vi "Create Connections.vi"(8 "error in (no error)":errorcluster, 11 "RT Data Cluster in":T1={"Timekeeper hdl"="", "clkDisc session"=variant, "Compiled Data"={"SyncMod?"=FALSE, "SyncMod"="", "ConnectionSettings"={"Mode"=enum."Generate sample clock", "pxitrig"=FALSE, "pfi0"=FALSE, "pfi1"=FALSE, "pfi2"=FALSE, "External Pin"=enum."PFI0", "Routes"=[]}, "TimeKeeper"="", "ScanOffset(%)"=0.0, "StartDelay(s)"=0, "Time Ref Settings"={"Time Reference"=enum."GPS", "Priority 1"=0, "Priority 2"=0, "IRIG type"=enum."IRIGB AM", "Terminal"="", "PPSSetTime"=FALSE, "Start Time"=timestamp(0 s since 1904-01-01)}, "FIFO Locations"={"BoardTime"=[], "Status"=[]}}, "OutputsData"=[], "OutputsFIFO"=refnum, "Scan Period"=0, "Timekeeper type"=enum."6683", "SyncMod type"=enum."6683", "SyncMod hdl"="", "Custom Device Name"=""} {"Compiled Data"."Time Ref Settings"."Priority 2" min=0 max=255; "Compiled Data"."Time Ref Settings"."Priority 1" min=0 max=255}) -> (0 "error out":errorcluster, 3 "RT Data Cluster out":T1={"Timekeeper hdl"="", "clkDisc session"=variant, "Compiled Data"={"SyncMod?"=FALSE, "SyncMod"="", "ConnectionSettings"={"Mode"=enum."Generate sample clock", "pxitrig"=FALSE, "pfi0"=FALSE, "pfi1"=FALSE, "pfi2"=FALSE, "External Pin"=enum."PFI0", "Routes"=[]}, "TimeKeeper"="", "ScanOffset(%)"=0.0, "StartDelay(s)"=0, "Time Ref Settings"={"Time Reference"=enum."GPS", "Priority 1"=0, "Priority 2"=0, "IRIG type"=enum."IRIGB AM", "Terminal"="", "PPSSetTime"=FALSE, "Start Time"=timestamp(0 s since 1904-01-01)}, "FIFO Locations"={"BoardTime"=[], "Status"=[]}}, "OutputsData"=[], "OutputsFIFO"=refnum, "Scan Period"=0, "Timekeeper type"=enum."6683", "SyncMod type"=enum."6683", "SyncMod hdl"="", "Custom Device Name"=""} {"Compiled Data"."Time Ref Settings"."Priority 2" min=0 max=255; "Compiled Data"."Time Ref Settings"."Priority 1" min=0 max=255})   [LabVIEW 2020, in "NI Synchronization Engine.lvlib"]
uses:
  NI Synchronization Engine.lvlib
  Timekeeper Route Pin.ctl
  <instrlib>/niSync/niSync.llb/niSync Create Clock (Frequency).vi
  <instrlib>/niSync/niSync.llb/niSync Initialize (Default).vi
  niveristand-synchronization-custom-device-2024/Source/Engine/mdevClkDisc.llb/_clkDisc_session.ctl
  Shared/Route.ctl
  Shared/NI Synchronization Shared.lvlib
  Shared/Routes.ctl
  Shared/External Pin.ctl
  Shared/Mode.ctl
  Shared/Connection Settings.ctl
  Shared/IRIG Type.ctl
  Shared/Time Ref Settings.ctl
  Shared/Compiled Data.ctl
  RT Data Cluster.ctl
  Shared/Time Reference.ctl
  timekeeper type.ctl
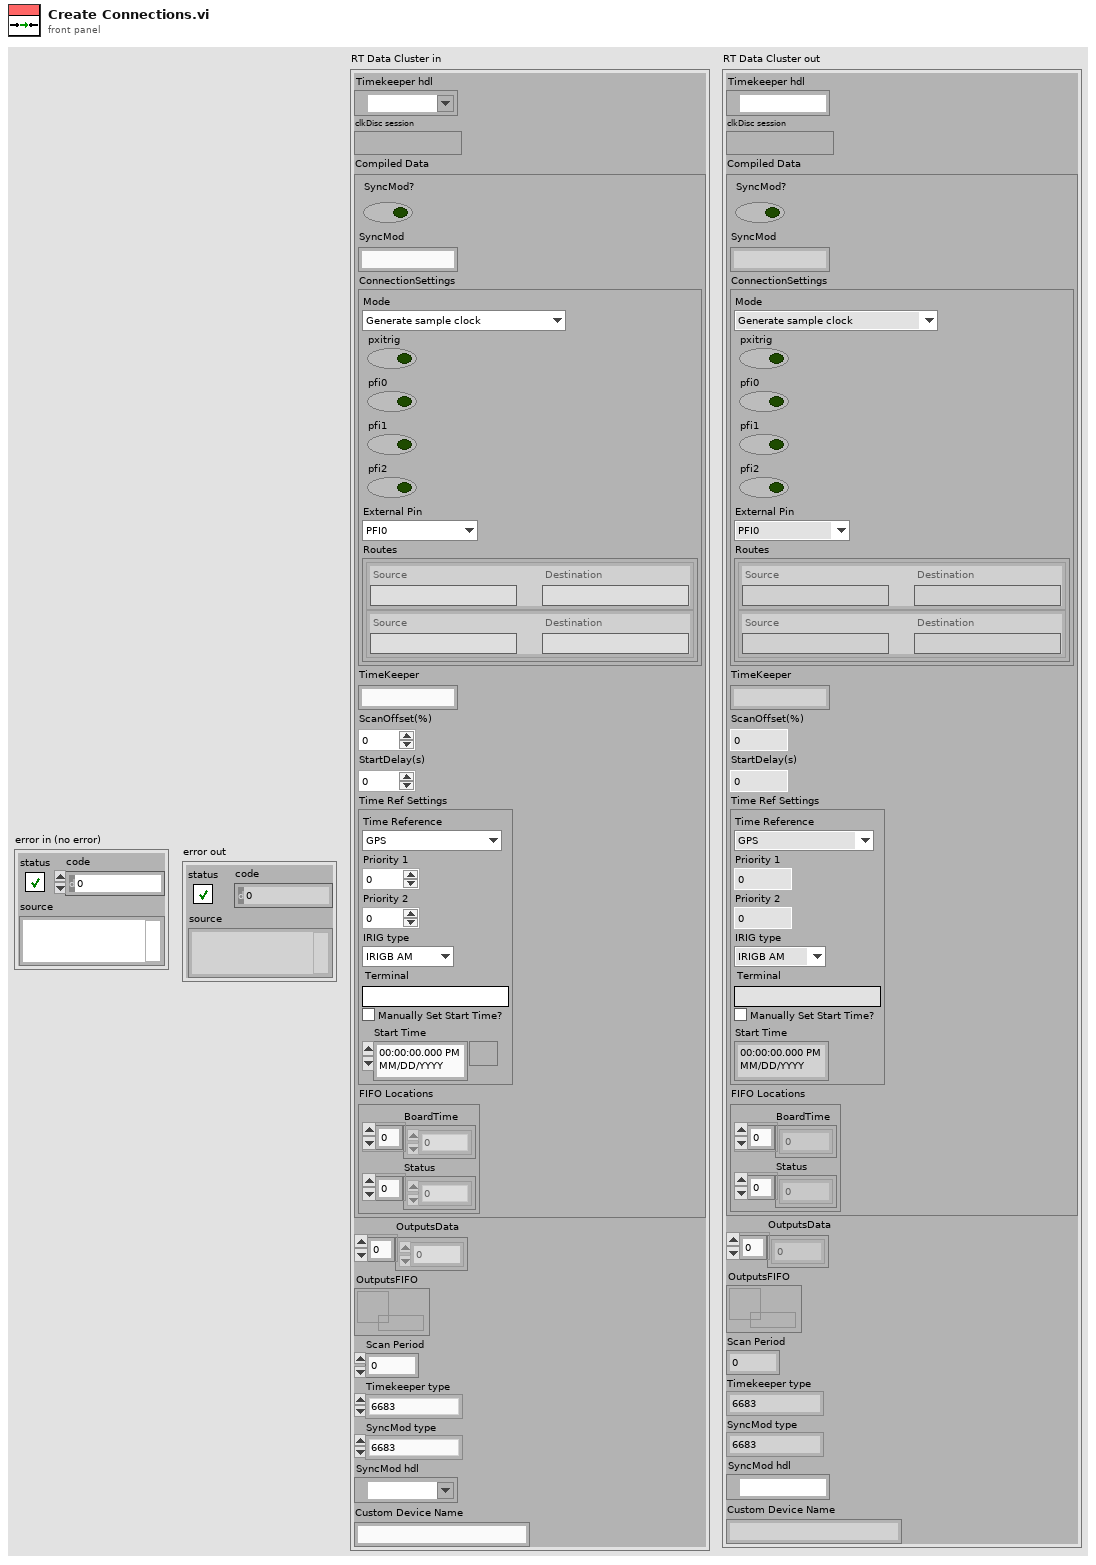
[diagram p1: front panel]
types:
  T1 = typedef "NI Synchronization Engine.lvlib/RT Data Cluster.ctl" = cluster{"Timekeeper hdl":refnum<k15>, "clkDisc session":T2, "Compiled Data":T3, "OutputsData":dbl[], "OutputsFIFO":refnum<k33>, "Scan Period":u32, "Timekeeper type":T12, "SyncMod type":T12, "SyncMod hdl":refnum<k15>, "Custom Device Name":string}
  T2 = typedef "_clkDisc_session.ctl" = variant
  T3 = typedef "NI Synchronization Shared.lvlib/Compiled Data.ctl" = cluster{"SyncMod?":bool, "SyncMod":string, "ConnectionSettings":T4, "TimeKeeper":string, "ScanOffset(%)":dbl, "StartDelay(s)":u16, "Time Ref Settings":T9, "FIFO Locations":cluster{"BoardTime":i32[], "Status":i32[]}}
  T4 = typedef "NI Synchronization Shared.lvlib/Connection Settings.ctl" = cluster{"Mode":T5, "pxitrig":bool, "pfi0":bool, "pfi1":bool, "pfi2":bool, "External Pin":T6, "Routes":T7}
  T5 = typedef "NI Synchronization Shared.lvlib/Mode.ctl" = enum16{"Generate sample clock", "Route sample clock out of chassis", "Route sample clock into chassis", "Custom routes"}
  T6 = typedef "NI Synchronization Shared.lvlib/External Pin.ctl" = enum16{"PFI0", "PFI1", "PFI2"}
  T7 = typedef "NI Synchronization Shared.lvlib/Routes.ctl" = T8[]
  T8 = typedef "NI Synchronization Shared.lvlib/Route.ctl" = cluster{"Source":string, "Destination":string}
  T9 = typedef "NI Synchronization Shared.lvlib/Time Ref Settings.ctl" = cluster{"Time Reference":T10, "Priority 1":i32, "Priority 2":i32, "IRIG type":T11, "Terminal":string, "PPSSetTime":bool, "Start Time":timestamp}
  T10 = typedef "NI Synchronization Shared.lvlib/Time Reference.ctl" = enum16{"GPS", "IRIG", "PPS", "1588 Ordinary Clock", "802.1AS", "PXI Chassis Clock", "Free Running (Internal)"}
  T11 = typedef "NI Synchronization Shared.lvlib/IRIG Type.ctl" = enum16{"IRIGB DC", "IRIGB AM"}
  T12 = typedef "NI Synchronization Engine.lvlib/timekeeper type.ctl" = enum16{"6683", "6683H", "6682", "6682H", "non-timekeeper", "timekeeper"}
  T13 = typedef "NI Synchronization Engine.lvlib/Timekeeper Route Pin.ctl" = enum16{"TTL0", "PFI0", "PFI1", "PFI2", "PXI_Clk10", "PXI_Clk10_In", "BoardClk", "ClkOut", "Oscillator"}
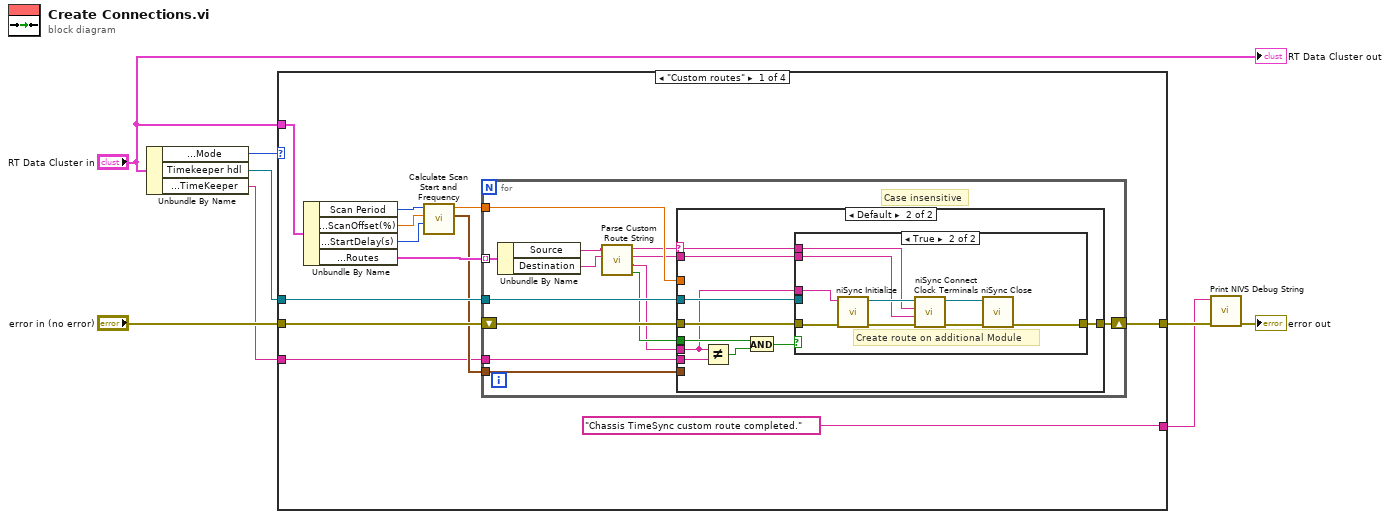
[diagram p0: block diagram]
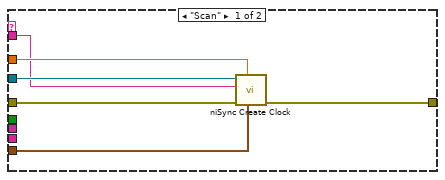
[diagram p2: hidden frame]
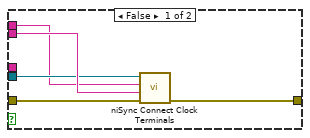
[diagram p3: hidden frame]
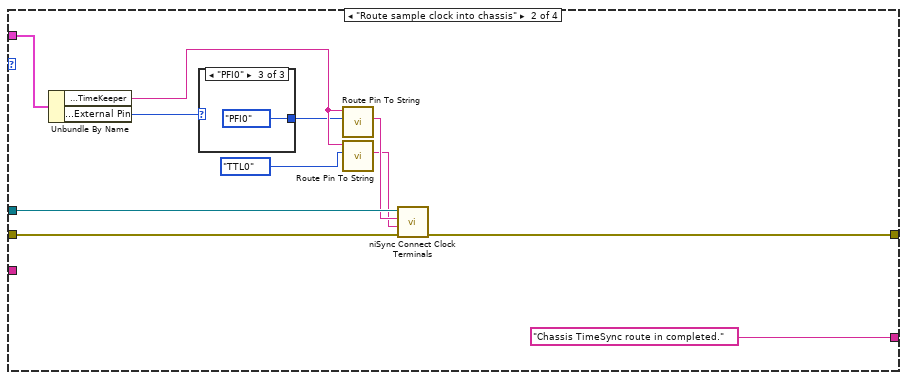
[diagram p4: hidden frame]
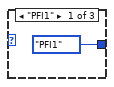
[diagram p5: hidden frame]
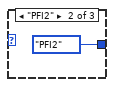
[diagram p6: hidden frame]
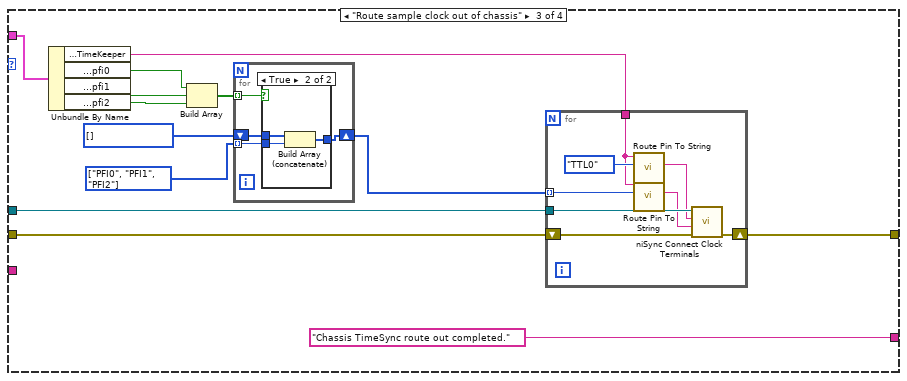
[diagram p7: hidden frame]
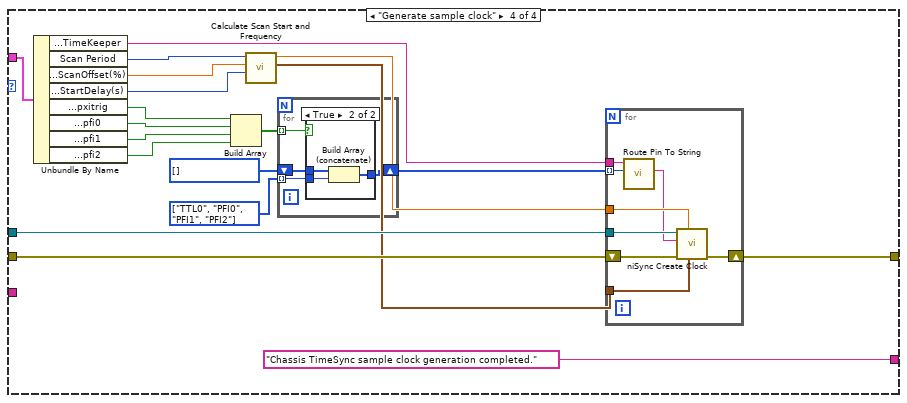
[diagram p9: hidden frame]
diagram:
  n1 = Unbundle By Name("RT Data Cluster in") -> ("Compiled Data.ConnectionSettings.Mode"=w8:T5, "Timekeeper hdl"=w7:refnum<k15>, "Compiled Data.TimeKeeper"=w1:string)
  n2 = case shown="\"Custom routes\"" w8 {
    tunnel: "error in (no error)" -> [w19 w68 w88 w122]
    tunnel: w7 -> [w16 w67 w87 w124]
    tunnel: "RT Data Cluster in" -> [w20 w74 w90 w121]
    tunnel: [w17 w72 w89 w125] -> w4
    tunnel: ["Chassis TimeSync custom route completed." "Chassis TimeSync route in completed." "Chassis TimeSync route out completed." "Chassis TimeSync sample clock generation completed."] -> w2
    tunnel: w1 -> [w10 _ _ _]
    frame "Custom routes" {
      n3 = Unbundle By Name(w20) -> ("Scan Period"=w15:u32, "Compiled Data.ScanOffset(%)"=w14:dbl, "Compiled Data.StartDelay(s)"=w13:u16, "Compiled Data.ConnectionSettings.Routes"=w18:T7)
      n4 = call "Calculate Scan Start and Frequency.vi"("Start delay (s)"=w13, "Start offset (fraction)"=w14, "Scan Period (uS)"=w15) -> ("Start time"=w11:timestamp, "Frequency"=w12:dbl)  [unwired: 7 in]
      n5 = for {
        shift-right: [w31] -> w17
        shift-left: w19 -> [w33]
        tunnel: w18 -> [w32] mode=indexing
        tunnel: w16 -> [w30]
        tunnel: w12 -> [w29]
        tunnel: w11 -> [w28]
        tunnel: w10 -> [w27]
        # "Case insensitive"
        n6 = Unbundle By Name(w32) -> ("Source"=w26:string, "Destination"=w25:string)
        n7 = call "Parse Custom Route String.vi"("Destination In"=w25, "Source In"=w26) -> ("Module?"=w24:bool, "Module Out"=w23:string, "Destination Out"=w21:string, "Source Out"=w22:string)  [unwired: 6 in]
        n8 = case shown="Default" w22 {
          selector: w22 -> [_ w45]
          tunnel: w33 -> [w39 w49]
          tunnel: w21 -> [w34 w48]
          tunnel: [w38 w47] -> w31
          tunnel: w30 -> [w37 w46]
          tunnel: w29 -> [w36 _]
          tunnel: w28 -> [w35 _]
          tunnel: w27 -> [_ w44]
          tunnel: w24 -> [_ w42]
          tunnel: w23 -> [_ w40]
          frame "Scan" {
            n9 = call-poly <instrlib>:"niSync Create Clock.vi"("start time"=w35, "frequency"=w36, "error in (no error)"=w39, "terminal"=w34, "instrument handle"=w37) -> ("error out"=w38:errorcluster)  [unwired: 3 in, 3 out]
          }
          frame Default {
            n10 = Not Equal?(x=w40, y=w44) -> (x != y?=w41:bool)
            n11 = And(x=w42, y=w41) -> (x .and. y?=w43:bool)
            n12 = case shown="True" w43 {
              tunnel: w49 -> [w54 w61]
              tunnel: w48 -> [w53 w57]
              tunnel: [w52 w55] -> w47
              tunnel: w46 -> [w51 _]
              tunnel: w45 -> [w50 w58]
              tunnel: w40 -> [_ w60]
              frame False {
                n13 = call <instrlib>:"niSync Connect Clock Terminals.vi"("error in (no error)"=w54, "destination terminal"=w53, "source terminal"=w50, "instrument handle"=w51) -> ("error out"=w52:errorcluster)  [unwired: 6 in, 1 out]
              }
              frame True {
                # "Create route on additional Module"
                n14 = call-poly <instrlib>:"niSync Initialize.vi"("error in (no error)"=w61, "resource name"=w60) -> ("error out"=w63:errorcluster, "instrument handle out"=w59:refnum<k15>)  [unwired: 8 in]
                n15 = call <instrlib>:"niSync Connect Clock Terminals.vi"("error in (no error)"=w63, "destination terminal"=w57, "source terminal"=w58, "instrument handle"=w59) -> ("error out"=w62:errorcluster, "instrument handle out"=w56:refnum<k15>)  [unwired: 6 in]
                n16 = call <instrlib>:"niSync Close.vi"("error in (no error)"=w62, "instrument handle"=w56) -> ("error out"=w55:errorcluster)  [unwired: 9 in]
              }
            }
          }
        }
      }
    }
    frame "Route sample clock into chassis" {
      n17 = Unbundle By Name(w74) -> ("Compiled Data.TimeKeeper"=w71:string, "Compiled Data.ConnectionSettings.External Pin"=w73:T6)
      n18 = case shown="\"PFI0\"" w73 {
        tunnel: [Timekeeper_Route_Pin."PFI1" ("Pin") Timekeeper_Route_Pin."PFI2" ("Pin") Timekeeper_Route_Pin."PFI0" ("Pin")] -> w69
        frame "PFI1" {
        }
        frame "PFI2" {
        }
        frame "PFI0" {
        }
      }
      n19 = call "Route Pin To String.vi"("Pin"=w69, "Module"=w71) -> ("String"=w66:string)  [unwired: 9 in]
      n20 = call "Route Pin To String.vi"("Pin"=Timekeeper_Route_Pin."TTL0", "Module"=w71) -> ("String"=w65:string)  [unwired: 9 in]
      n21 = call <instrlib>:"niSync Connect Clock Terminals.vi"("error in (no error)"=w68, "destination terminal"=w65, "source terminal"=w66, "instrument handle"=w67) -> ("error out"=w72:errorcluster)  [unwired: 6 in, 1 out]
    }
    frame "Route sample clock out of chassis" {
      w80 = T13[] [enum."PFI0", enum."PFI1", enum."PFI2"] items=["TTL0", "PFI0", "PFI1", "PFI2", "PXI_Clk10", "PXI_Clk10_In", "BoardClk", "ClkOut", "Oscillator"]
      w81 = T13[] [] items=["TTL0", "PFI0", "PFI1", "PFI2", "PXI_Clk10", "PXI_Clk10_In", "BoardClk", "ClkOut", "Oscillator"]
      n22 = Unbundle By Name(w90) -> ("Compiled Data.TimeKeeper"=w86:string, "Compiled Data.ConnectionSettings.pfi0"=w85:bool, "Compiled Data.ConnectionSettings.pfi1"=w84:bool, "Compiled Data.ConnectionSettings.pfi2"=w83:bool)
      n23 = Build Array(w85, w84, w83) -> (w82:bool[])
      n24 = for {
        tunnel: w82 -> [w94] mode=indexing
        shift-right: [w91] -> w79
        shift-left: w81 -> [w93]
        tunnel: w80 -> [w92] mode=indexing
        n25 = case shown="True" w94 {
          tunnel: w93 -> [w95 w98]
          tunnel: w92 -> [_ w97]
          tunnel: [w95 w96] -> w91
          frame False {
          }
          frame True {
            n26 = Build Array (concatenate)(w98, w97) -> (w96:T13[])
          }
        }
      }
      n27 = for {
        tunnel: w87 -> [w104]
        shift-right: [w106] -> w89
        shift-left: w88 -> [w105]
        tunnel: w86 -> [w101]
        tunnel: w79 -> [w99] mode=indexing
        n28 = call "Route Pin To String.vi"("Pin"=Timekeeper_Route_Pin."TTL0", "Module"=w101) -> ("String"=w103:string)  [unwired: 9 in]
        n29 = call "Route Pin To String.vi"("Pin"=w99, "Module"=w101) -> ("String"=w100:string)  [unwired: 9 in]
        n30 = call <instrlib>:"niSync Connect Clock Terminals.vi"("error in (no error)"=w105, "destination terminal"=w100, "source terminal"=w103, "instrument handle"=w104) -> ("error out"=w106:errorcluster)  [unwired: 6 in, 1 out]
      }
    }
    frame "Generate sample clock" {
      w113 = T13[] [enum."TTL0", enum."PFI0", enum."PFI1", enum."PFI2"] items=["TTL0", "PFI0", "PFI1", "PFI2", "PXI_Clk10", "PXI_Clk10_In", "BoardClk", "ClkOut", "Oscillator"]
      w114 = T13[] [] items=["TTL0", "PFI0", "PFI1", "PFI2", "PXI_Clk10", "PXI_Clk10_In", "BoardClk", "ClkOut", "Oscillator"]
      n31 = Unbundle By Name(w121) -> ("Compiled Data.TimeKeeper"=w111:string, "Scan Period"=w120:u32, "Compiled Data.ScanOffset(%)"=w119:dbl, "Compiled Data.StartDelay(s)"=w118:u16, "Compiled Data.ConnectionSettings.pxitrig"=w110:bool, "Compiled Data.ConnectionSettings.pfi0"=w109:bool, "Compiled Data.ConnectionSettings.pfi1"=w108:bool, "Compiled Data.ConnectionSettings.pfi2"=w107:bool)
      n32 = Build Array(w110, w109, w108, w107) -> (w115:bool[])
      n33 = call "Calculate Scan Start and Frequency.vi"("Start delay (s)"=w118, "Start offset (fraction)"=w119, "Scan Period (uS)"=w120) -> ("Start time"=w116:timestamp, "Frequency"=w117:dbl)  [unwired: 7 in]
      n34 = for {
        tunnel: w115 -> [w129] mode=indexing
        shift-right: [w126] -> w112
        shift-left: w114 -> [w128]
        tunnel: w113 -> [w127] mode=indexing
        n35 = case shown="True" w129 {
          tunnel: w128 -> [w130 w133]
          tunnel: w127 -> [_ w132]
          tunnel: [w130 w131] -> w126
          frame False {
          }
          frame True {
            n36 = Build Array (concatenate)(w133, w132) -> (w131:T13[])
          }
        }
      }
      n37 = for {
        shift-right: [w140] -> w125
        shift-left: w122 -> [w141]
        tunnel: w124 -> [w139]
        tunnel: w117 -> [w138]
        tunnel: w116 -> [w137]
        tunnel: w112 -> [w136] mode=indexing
        tunnel: w111 -> [w134]
        n38 = call "Route Pin To String.vi"("Pin"=w136, "Module"=w134) -> ("String"=w135:string)  [unwired: 9 in]
        n39 = call-poly <instrlib>:"niSync Create Clock.vi"("start time"=w137, "frequency"=w138, "error in (no error)"=w141, "terminal"=w135, "instrument handle"=w139) -> ("error out"=w140:errorcluster)  [unwired: 3 in, 3 out]
      }
    }
  }
  n40 = call "Print NIVS Debug String.vi"("error in (no error)"=w4, "Debug String"=w2) -> ("error out"=→"error out":errorcluster)  [unwired: 8 in]
  "RT Data Cluster out" <- "RT Data Cluster in"
